vi "Empty Array.vi"() -> (0 "error out":errorcluster)   [LabVIEW 2017, in "Transparent Assertions.Tests.lvlib" / "Assert Count.lvlib"]
uses:
  Assert Count.lvlib
  src/Transparent Assertions/Transparent Assertions.lvlib
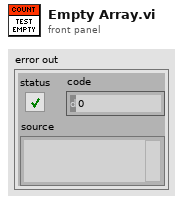
[diagram p1: front panel]
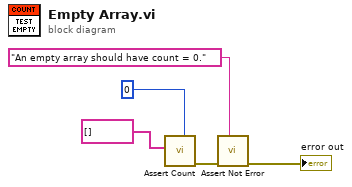
[diagram p0: block diagram]
diagram:
  n1 = call "Assert Count.vi"("Expected"=0, "Haystack"=string[] []) -> ("error out"=w3:errorcluster)  [unwired: 9 in]
  n2 = call "Assert Not Error.vi"("Message (\"\")"="An empty array should have count = 0." ("Message (\"\")"), "error in (no error)"=w3) -> ("error out"=→"error out":errorcluster)  [unwired: 9 in]
